vi "Load IOPanel.vi"(8 "error in (no error)":errorcluster, 11 "MPC_AutoInspection in":refnum<class "MPC_AutoInspection.lvclass">) -> (0 "error out":errorcluster, 2 "This VI":refnum<vi>, 3 "MPC_AutoInspection out":refnum<class "MPC_AutoInspection.lvclass">)   [LabVIEW 2019, in "MPC_AutoInspection.lvclass"]
uses:
  MPC_AutoInspection.lvclass
  Function/IO Folder/IO_VI/IOCtrl/Ctrl/IO Card_Type.ctl
  Function/IO Folder/IO_Class/IOCard.lvclass
  Function/IO Folder/IO_Class/IOCard.lvclass/IOCard.ctl
panel:
  in  "Tab Control":enum32{"Page 1", "Page 2"}(tab)
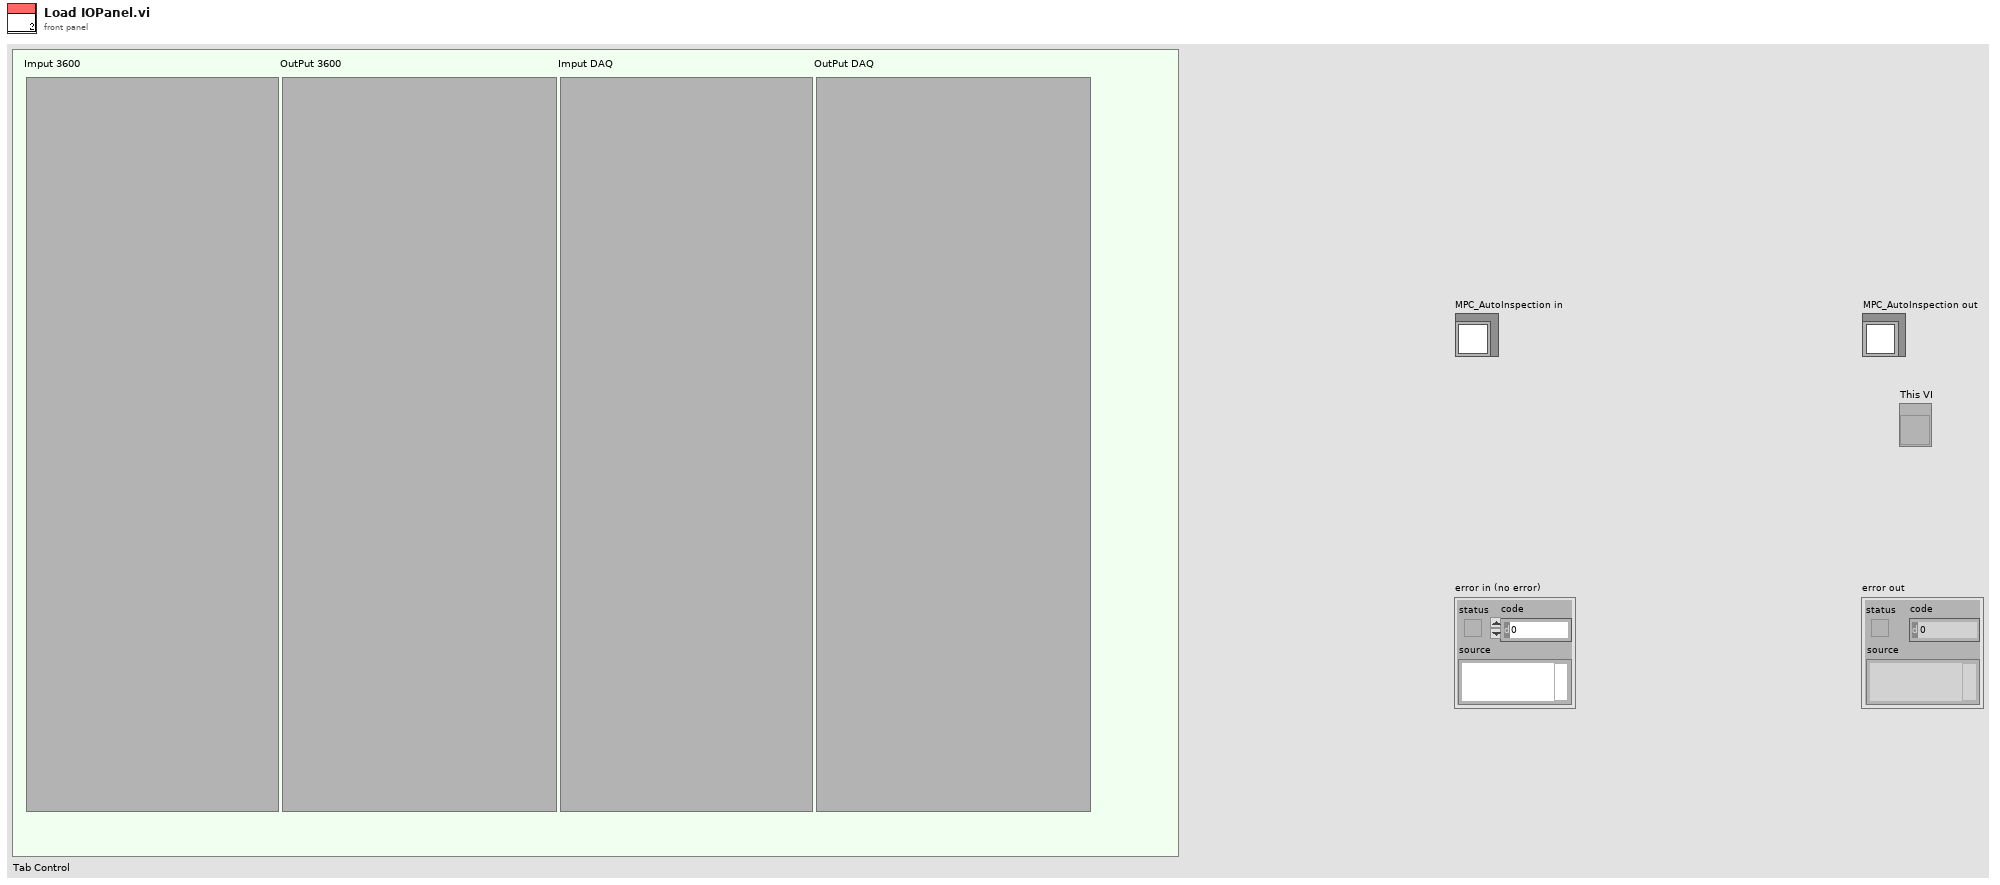
[diagram p1: front panel]
types:
  T1 = typedef "IO Card_Type.ctl" = enum16{"None", "Unidaq32", "6480", "2410C-64", "Zan", "DMC1000B", "16InOut", "Robot", "DMC3600"}
  T2 = cluster{"IO Card Type":T1, "IOType":enum16{"Input", "Output"}, "CardNumber":i32, "ConnectAct":bool, "IP":string}
  T3 = typedef "LVPointTypeDef.ctl" = cluster{"Horizontal":i16, "Vertical":i16}
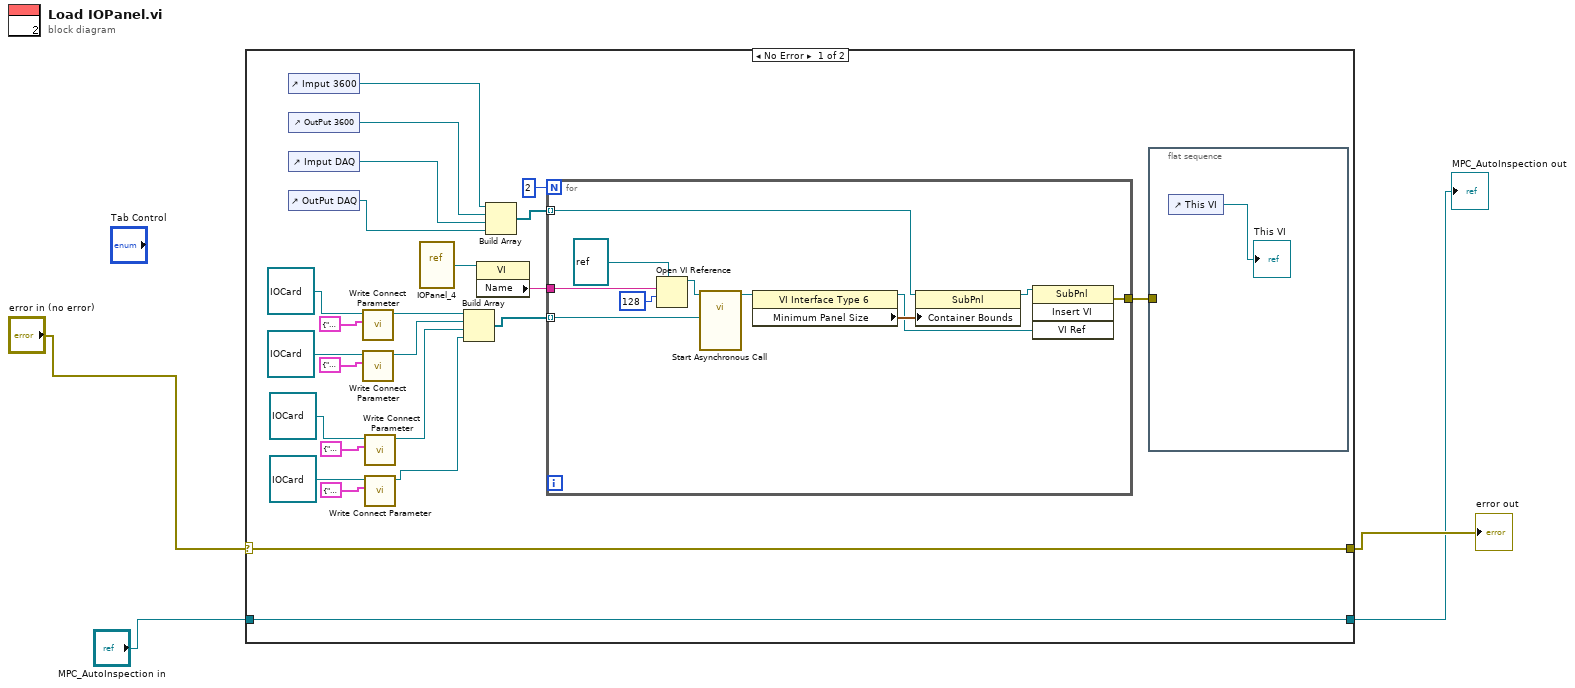
[diagram p0: block diagram]
diagram:
  n1 = case shown="No Error" "error in (no error)" {
    selector: "error in (no error)" -> [w22 w42]
    tunnel: [w22 w42] -> w3
    tunnel: [w21 w41] -> w2
    tunnel: "MPC_AutoInspection in" -> [w21 w41]
    frame No Error {
      n2 = control-ref of="Imput 3600"() -> (w14:refnum<vi>)
      n3 = control-ref of="OutPut 3600"() -> (w13:refnum<vi>)
      n4 = control-ref of="Imput DAQ"() -> (w12:refnum<vi>)
      n5 = control-ref of="OutPut DAQ"() -> (w11:refnum<vi>)
      n6 = call "Write Connect Parameter.vi"("Connect Parameter"=T2 {"IO Card Type"=enum."DMC3600", "IOType"=enum."Input", "CardNumber"=0, "ConnectAct"=TRUE, "IP"=""}, "IOCard in"=refnum<class "IOCard.lvclass"> refnum ("IOCard.lvclass")) -> ("IOCard out"=w19:refnum<class "IOCard.lvclass">)  [unwired: 8 in, 1 out]
      n7 = call "Write Connect Parameter.vi"("Connect Parameter"=T2 {"IO Card Type"=enum."DMC3600", "IOType"=enum."Output", "CardNumber"=0, "ConnectAct"=FALSE, "IP"=""}, "IOCard in"=refnum<class "IOCard.lvclass"> refnum ("IOCard.lvclass")) -> ("IOCard out"=w17:refnum<class "IOCard.lvclass">)  [unwired: 8 in, 1 out]
      n8 = call "Write Connect Parameter.vi"("Connect Parameter"=T2 {"IO Card Type"=enum."Unidaq32", "IOType"=enum."Input", "CardNumber"=0, "ConnectAct"=TRUE, "IP"=""}, "IOCard in"=refnum<class "IOCard.lvclass"> refnum ("IOCard.lvclass")) -> ("IOCard out"=w6:refnum<class "IOCard.lvclass">)  [unwired: 8 in, 1 out]
      n9 = call "Write Connect Parameter.vi"("Connect Parameter"=T2 {"IO Card Type"=enum."Unidaq32", "IOType"=enum."Output", "CardNumber"=0, "ConnectAct"=FALSE, "IP"=""}, "IOCard in"=refnum<class "IOCard.lvclass"> refnum ("IOCard.lvclass")) -> ("IOCard out"=w5:refnum<class "IOCard.lvclass">)  [unwired: 8 in, 1 out]
      n10 = vi-ref "IOPanel_4.vi"() -> (w16:refnum<vi>)
      n11 = Build Array(w19, w17, w6, w5) -> (w18:refnum<class "IOCard.lvclass">[])
      n12 = property class="VI"(reference=w16) -> ("Name"=w25:string)  [unwired: 1 in, 2 out]
      n13 = Build Array(w14, w13, w12, w11) -> (w23:refnum<vi>[])
      n14 = for {
        N: 2 -> [_]
        tunnel: w25 -> [w40]
        tunnel: w18 -> [w36] mode=indexing
        tunnel: w23 -> [w33] mode=indexing
        tunnel: [w35] -> w20
        n15 = Open VI Reference(type specifier VI Refnum (for type only)=refnum<vi> refnum, vi path=w40, options=128) -> (vi reference=w37:refnum<vi>)  [unwired: 3 in, 1 out]
        n16 = call-by-ref "Start Asynchronous Call"(reference=w37, "IOCard In"=w36) -> (reference out=w34:refnum<vi>)  [unwired: 12 in, 1 out]
        n17 = property class="VI Interface Type 6"(reference=w34) -> (reference out=w30:refnum<vi>, "Minimum Panel Size"=w31:T3)  [unwired: 1 in, 1 out]
        n18 = property class="SubPnl"(reference=w33, "Container Bounds"=w31) -> (reference out=w32:refnum<vi>)  [unwired: 1 in, 1 out]
        n19 = invoke class="SubPnl" method="Insert VI"(reference=w32, "VI Ref"=w30) -> (error out=w35:errorcluster)  [unwired: 2 in, 3 out]
      }
      n20 = flat-sequence {
        tunnel: w20 -> [_]
        frame #0 {
          n21 = control-ref of="This VI"() -> (→"This VI":refnum<vi>)
        }
      }
    }
    frame Error {
    }
  }
  "error out" <- w3
  "MPC_AutoInspection out" <- w2
